vi "Read SDI Address.vi"(8 "error in (no error)":errorcluster, 11 "H3611i in":refnum<class "H3611i.lvclass">) -> (0 "error out":errorcluster, 2 "SDI Address":string, 3 "H3611i out":refnum<class "H3611i.lvclass">)   [LabVIEW 2017, in "Sensors.lvlib" / "H3611i.lvclass"]
uses:
  H3611i.lvclass
  H3611i.lvclass/H3611i.ctl
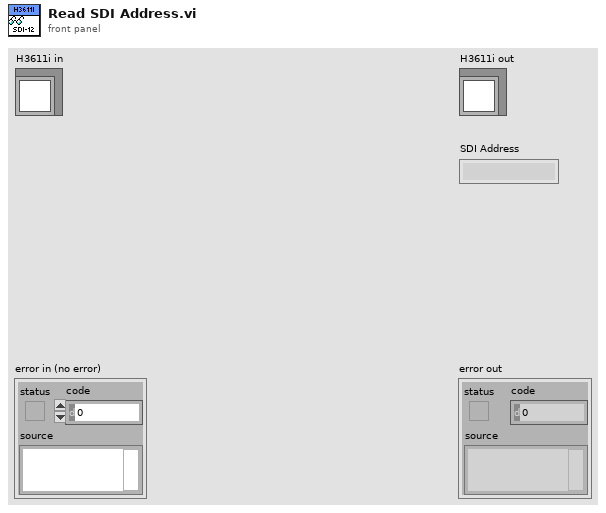
[diagram p1: front panel]
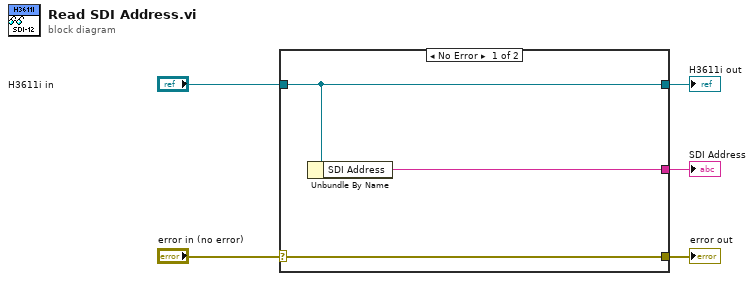
[diagram p0: block diagram]
diagram:
  n1 = case shown="No Error" "error in (no error)" {
    selector: "error in (no error)" -> [w8 w9]
    tunnel: [w8 w9] -> w4
    tunnel: [w7 w10] -> w2
    tunnel: "H3611i in" -> [w7 w10]
    tunnel: [w6 _] -> w1
    frame No Error {
      n2 = Unbundle By Name(w7) -> ("SDI Address"=w6:string)
    }
    frame Error {
    }
  }
  "error out" <- w4
  "H3611i out" <- w2
  "SDI Address" <- w1
